vi "Emphasize Color.vi"(2 "error in 2 (no error)":errorcluster, 3 "Color":i8, 4 "Image Dst":T1, 5 "Image Src":T1) -> (0 "error out":errorcluster, 1 "Image Out":T1)   [LabVIEW 2009, in "ImageProcessing.lvlib"]
doc: "Output is a grayscaled image calculated as\n (255*X)/(R+G+B) \nwhere X is R, G or B depending on what number is showsen in color (0 = R, 1 = G, 2 = B)."
uses:
  ImageProcessing.lvlib
  <vilib>/vision/Image Controls.llb/IMAQ Image.ctl
  <vilib>/Analysis/Matrix/Numeric/Conversions/Matrix To Array - RM.vi
  <vilib>/Analysis/Matrix/Numeric/Add/Add - RM,RM.vi
  <vilib>/Analysis/Matrix/Numeric/Multiply/Multiply - RM,R.vi
  <vilib>/Analysis/Matrix/Numeric/Conversions/Array To Matrix - RA2.vi
  <vilib>/vision/NI_Vision_Development_Module.lvlib
  <vilib>/Analysis/Matrix/NI_Matrix.lvlib
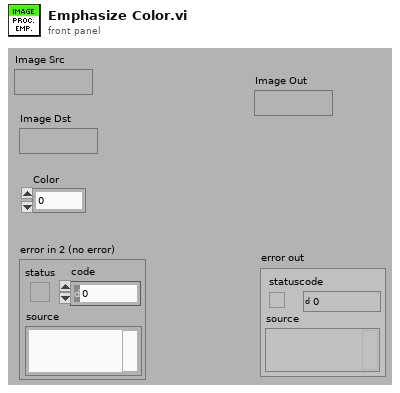
[diagram p1: front panel]
types:
  T1 = typedef "IMAQ Image.ctl" = refnum<image>
  T2 = typedef "NI_Matrix.lvlib/RealMatrix.ctl" = dbl[][]
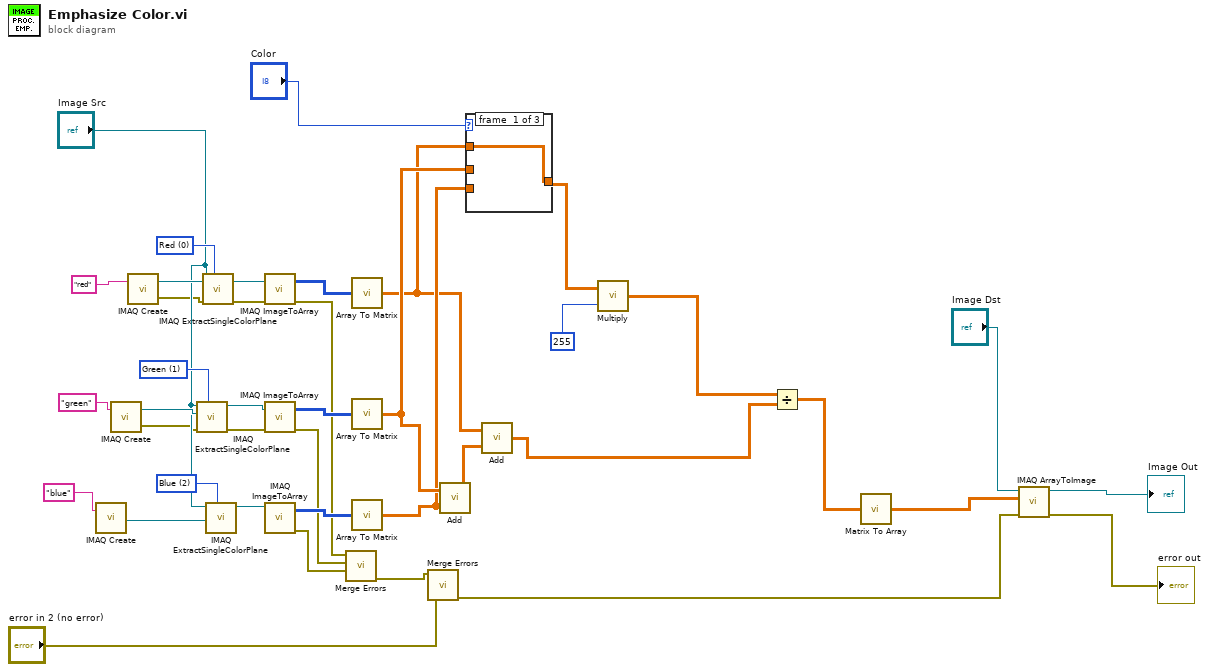
[diagram p0: block diagram]
diagram:
  w32 = 2 items=["Red", "Green", "Blue", "Hue", "Saturation", "Luminance", "Value", "Intensity"] ("Color Plane")
  w33 = 1 items=["Red", "Green", "Blue", "Hue", "Saturation", "Luminance", "Value", "Intensity"] ("Color Plane")
  w34 = 0 items=["Red", "Green", "Blue", "Hue", "Saturation", "Luminance", "Value", "Intensity"] ("Color Plane")
  n1 = call "IMAQ Create"("Image Name"="blue") -> ("New Image"=w35:T1)  [unwired: 3 in, 2 out]
  n2 = call "IMAQ Create"("Image Name"="green") -> ("New Image"=w36:T1, "error out"=w11:errorcluster)  [unwired: 3 in, 1 out]
  n3 = call "IMAQ Create"("Image Name"="red") -> ("New Image"=w37:T1, "error out"=w13:errorcluster)  [unwired: 3 in, 1 out]
  n4 = call "IMAQ ExtractSingleColorPlane"("Color Plane"=w33, "error in (no error)"=w11, "Image Dst"=w36, "Image Src"="Image Src") -> ("error out"=w10:errorcluster, "Image Dst Out"=w3:T1)  [unwired: 6 in]
  n5 = call "IMAQ ExtractSingleColorPlane"("Color Plane"=w34, "error in (no error)"=w13, "Image Dst"=w37, "Image Src"="Image Src") -> ("error out"=w12:errorcluster, "Image Dst Out"=w2:T1)  [unwired: 6 in]
  n6 = call "IMAQ ExtractSingleColorPlane"("Color Plane"=w32, "Image Dst"=w35, "Image Src"="Image Src") -> ("Image Dst Out"=w31:T1)  [unwired: 7 in, 1 out]
  n7 = call "IMAQ ImageToArray"("error in (no error)"=w12, "Image"=w2) -> ("error out"=w9:errorcluster, "Image Pixels (U8)"=w30:u8[][])  [unwired: 2 in, 3 out]
  n8 = call "IMAQ ImageToArray"("error in (no error)"=w10, "Image"=w3) -> ("error out"=w8:errorcluster, "Image Pixels (U8)"=w29:u8[][])  [unwired: 2 in, 3 out]
  n9 = call "IMAQ ImageToArray"("Image"=w31) -> ("error out"=w7:errorcluster, "Image Pixels (U8)"=w28:u8[][])  [unwired: 3 in, 3 out]
  n10 = call <vilib>:"Merge Errors.vi"("error in 3 (no error)"=w7, "error in 2 (no error)"=w8, "error in 1 (no error)"=w9) -> ("error out"=w5:errorcluster)  [unwired: 4 in]
  n11 = call-poly <vilib>:"Array To Matrix.vi"("Real 2D Array"=w30) -> ("Real Matrix"=w16:T2)
  n12 = call-poly <vilib>:"Array To Matrix.vi"("Real 2D Array"=w29) -> ("Real Matrix"=w19:T2)
  n13 = call-poly <vilib>:"Array To Matrix.vi"("Real 2D Array"=w28) -> ("Real Matrix"=w18:T2)
  n14 = call <vilib>:"Merge Errors.vi"("error in 2 (no error)"="error in 2 (no error)", "error in 1 (no error)"=w5) -> ("error out"=w6:errorcluster)  [unwired: 5 in]
  n15 = call-poly <vilib>:"Add.vi"("Real Matrix B"=w18, "Real Matrix A"=w19) -> ("A + B"=w27:T2)
  n16 = case shown="..0" "Color" {
    tunnel: w16 -> [w41 _ _]
    tunnel: w19 -> [_ w42 _]
    tunnel: w18 -> [_ _ w43]
    tunnel: [w41 w42 w43] -> w15
    frame #0 {
    }
    frame #1 {
    }
    frame #2 {
    }
  }
  n17 = call-poly <vilib>:"Add.vi"("Real Matrix B"=w27, "Real Matrix A"=w16) -> ("A + B"=w25:T2)
  n18 = call-poly <vilib>:"Multiply.vi"("Real Scalar c"=255, "Real Matrix A"=w15) -> ("A * c"=w24:T2)
  n19 = Divide(x=w24, y=w25) -> (x/y=w23:T2)
  n20 = call-poly <vilib>:"Matrix To Array.vi"("Real Matrix"=w23) -> ("Real 2D Array"=w22:dbl[][])
  n21 = call "IMAQ ArrayToImage"("error in (no error)"=w6, "Image Pixels (U8)"=w22, "Image"="Image Dst") -> ("error out"=→"error out":errorcluster, "Image Out"=→"Image Out":T1)  [unwired: 7 in]
